vi "Read port broadcast.vi"(8 "error in (no error)":errorcluster, 11 "Kasli Wrapper 2 in":refnum<class "Kasli Wrapper 2.0.lvclass">=refnum) -> (0 "error out":errorcluster, 2 "port broadcast":u32, 3 "Kasli Wrapper 2 out":refnum<class "Kasli Wrapper 2.0.lvclass">)   [LabVIEW 2020, in "CIRCUS_uServices.lvlib" / "Kasli Wrapper 2.0.lvlib" / "Kasli Wrapper 2.0.lvclass"]
uses:
  Kasli Wrapper 2.0.lvclass
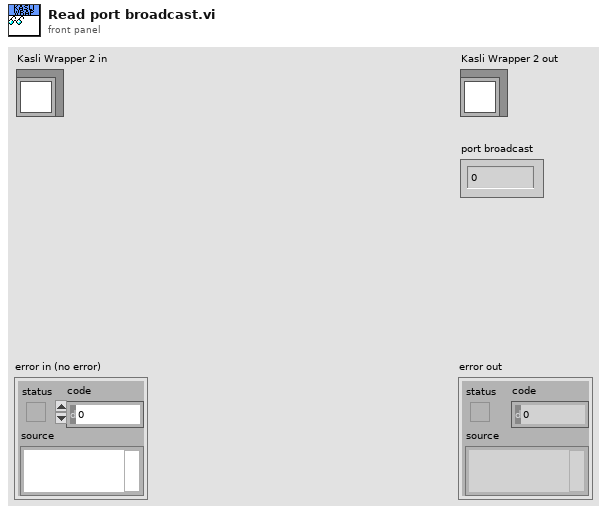
[diagram p1: front panel]
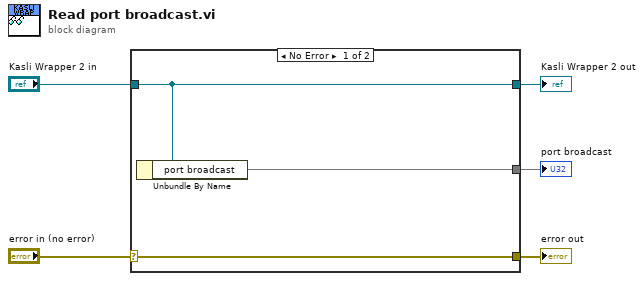
[diagram p0: block diagram]
diagram:
  n1 = case shown="No Error" "error in (no error)" {
    selector: "error in (no error)" -> [w8 w9]
    tunnel: [w8 w9] -> w4
    tunnel: [w7 w10] -> w2
    tunnel: "Kasli Wrapper 2 in" -> [w7 w10]
    tunnel: [w6 _] -> w1
    frame No Error {
      n2 = Unbundle By Name(w7) -> ("port broadcast"=w6)
    }
    frame Error {
    }
  }
  "error out" <- w4
  "Kasli Wrapper 2 out" <- w2
  "port broadcast" <- w1
